vi "FXP NILIA_CIC_Stage.vi"(8 "decimate factor":i16, 9 "New Data":bool, 11 "input":i64) -> (1 "Data Ready":bool, 3 "output":i64)   [LabVIEW 2012]
uses:
  <vilib>/rvi/Emulation/niFpgaSctlEmulationGetInTimedLoop.vi
  <vilib>/rvi/Emulation/niFpgaSctlEmulationGlobalWrite.vi
panel:
  in  "count":i16
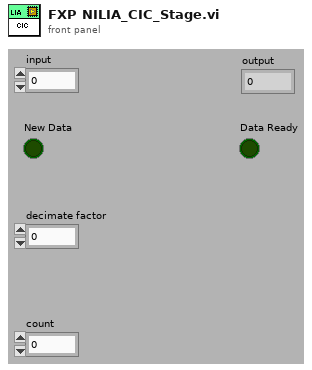
[diagram p1: front panel]
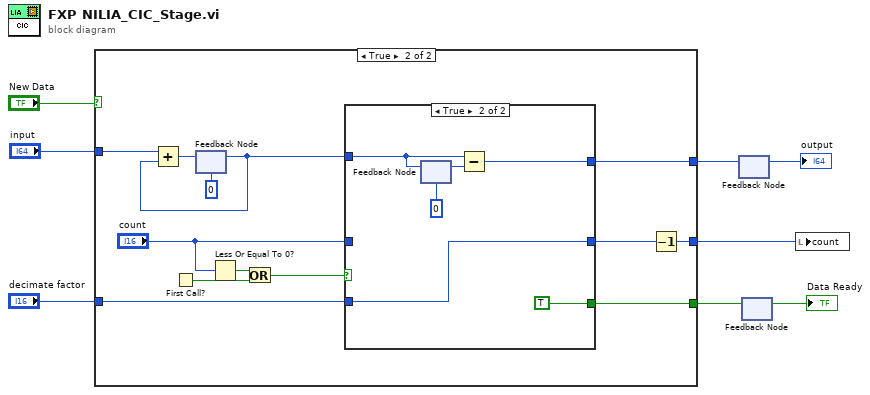
[diagram p0: block diagram]
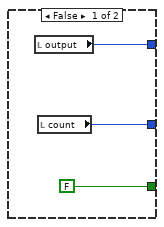
[diagram p2: hidden frame]
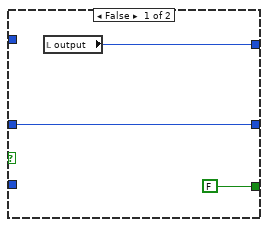
[diagram p3: hidden frame]
diagram:
  n1 = case shown="True" "New Data" {
    tunnel: [w10 w24] -> w4
    tunnel: "decimate factor" -> [_ w23]
    tunnel: [w11 w21] -> w7
    tunnel: "input" -> [_ w15]
    tunnel: [FALSE ("Data Ready") w14] -> w2
    frame False {
      n2 = local read "output"() -> (w10:i64)
      n3 = local read "count"() -> (w11:i16)
    }
    frame True {
      n4 = First Call?() -> (First Call?: T/F=w19:bool)
      n5 = feedback #1(i64 0) -> (w12:i64)
      n6 = Add(x=w15, y=w12) -> (x+y=w13:i64)
      n7 = feedback-in #1(w13) -> ()
      n8 = Less Or Equal To 0?(x="count") -> (x <= 0?=w20:bool)
      n9 = Or(x=w20, y=w19) -> (x .or. y?=w18:bool)
      n10 = case shown="True" w18 {
        tunnel: w12 -> [_ w29]
        tunnel: [w26 w28] -> w24
        tunnel: "count" -> [w27 _]
        tunnel: [w27 w33] -> w22
        tunnel: w23 -> [_ w33]
        tunnel: [FALSE ("Data Ready") TRUE ("Data Ready")] -> w14
        frame False {
          n11 = local read "output"() -> (w26:i64)
        }
        frame True {
          n12 = feedback-in #2(w29) -> ()
          n13 = feedback #2(i64 0) -> (w32:i64)
          n14 = Subtract(x=w29, y=w32) -> (x-y=w28:i64)
        }
      }
      n15 = Decrement(x=w22) -> (x-1=w21:i16)
    }
  }
  n16 = feedback-in #3(w4) -> ()
  n17 = feedback #3() -> (→"output":i64)  [unwired: 1 in]
  n18 = feedback-in #4(w2) -> ()
  n19 = feedback #4() -> (→"Data Ready":bool)  [unwired: 1 in]
  n20 = local write "count"(w7) -> ()
